vi "RSW_array.vi"() -> ()   [LabVIEW 2015]
doc: "Reading an ini file, sorting using an array, writing sorted data to an ini file"
uses:
  <vilib>/Utility/config.llb/Read Key (String).vi
  <vilib>/Utility/config.llb/Write Key (String).vi
  <vilib>/Utility/config.llb/Write Key (Double).vi
  <vilib>/Utility/config.llb/NI_LVConfig.lvlib
panel:
  out "Sorted":T1(array[cluster])
  out "Unsorted":T1(array[cluster])
  out "error out":errorcluster
  in  "Sorted ini file":path
  in  "The path of the ini file":path
  in  "Cluster":T2
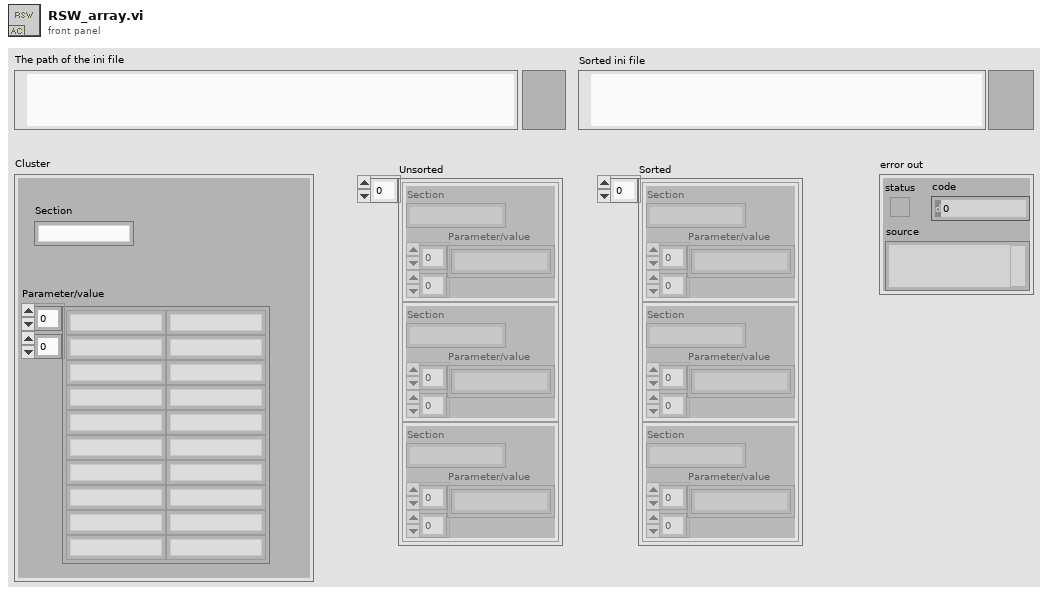
[diagram p1: front panel]
types:
  T1 = cluster{"Section":string, "Parameter/value":string[][]}[]
  T2 = cluster{"Section":string, "Parameter/value":string[][]}
  T3 = typedef "NI_LVConfig.lvlib/Config Data RefNum.ctl" = refnum<k1>
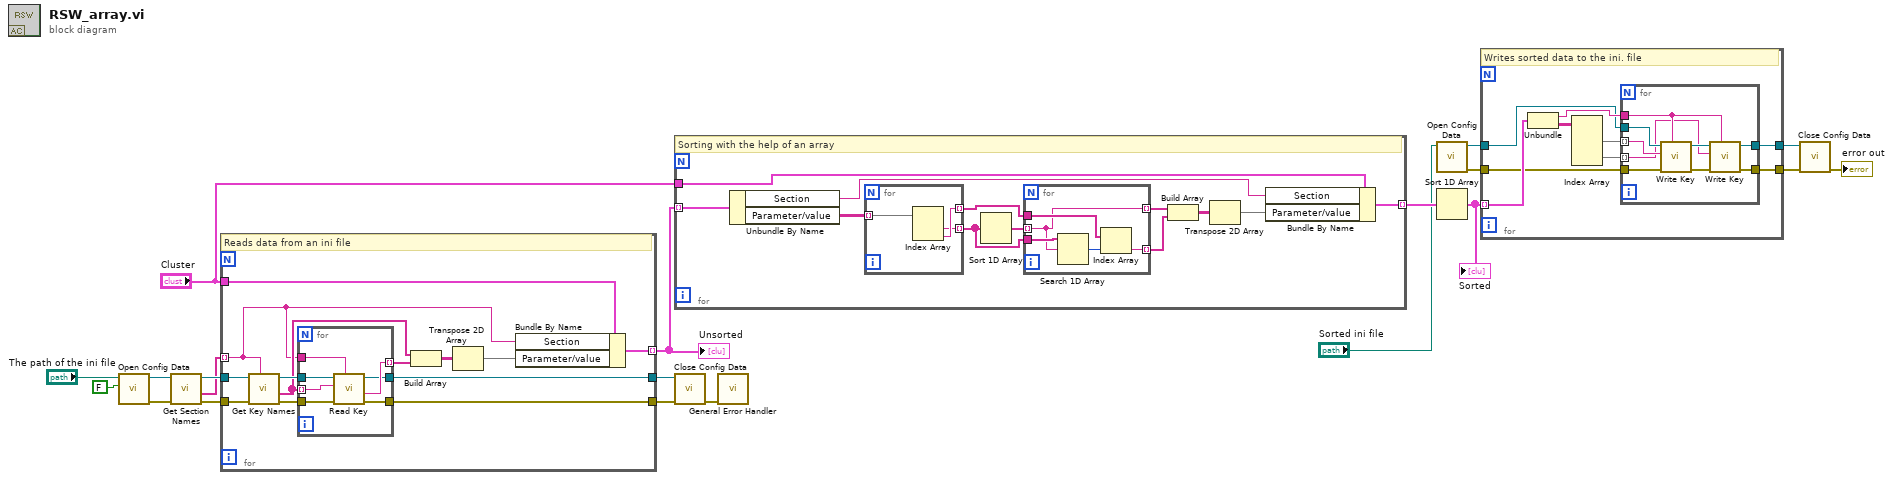
[diagram p0: block diagram]
diagram:
  n1 = call <vilib>:"Open Config Data.vi"("create file if necessary (T)"=FALSE, "configuration file path"="The path of the ini file") -> ("error out"=w19:errorcluster, "refnum"=w20:T3)  [unwired: 7 in, 1 out]
  n2 = call <vilib>:"Get Section Names.vi"("error in (no error)"=w19, "refnum"=w20) -> ("error out"=w17:errorcluster, "section names"=w16:string[], "refnum out"=w18:T3)  [unwired: 7 in]
  n3 = for {
    tunnel: w16 -> [w26] mode=indexing
    tunnel: w18 -> [w32]
    tunnel: w17 -> [w33]
    tunnel: [w25] -> w2 mode=indexing
    tunnel: "Cluster" -> [w24]
    tunnel: [w22] -> w9
    tunnel: [w21] -> w10
    # "Reads data from an ini file"
    n4 = call <vilib>:"Get Key Names.vi"("section"=w26, "error in (no error)"=w33, "refnum"=w32) -> ("error out"=w31:errorcluster, "key names"=w29:string[], "refnum out"=w30:T3)  [unwired: 5 in, 1 out]
    n5 = for {
      tunnel: w26 -> [w40]
      tunnel: w29 -> [w39] mode=indexing
      tunnel: w30 -> [w38]
      tunnel: w31 -> [w37]
      tunnel: [w36] -> w28 mode=indexing
      tunnel: [w35] -> w22
      tunnel: [w34] -> w21
      n6 = call-poly <vilib>:"Read Key.vi"("section"=w40, "error in (no error)"=w37, "key"=w39, "refnum"=w38) -> ("error out"=w35:errorcluster, "value"=w36:string, "refnum out"=w34:T3)  [unwired: 4 in, 1 out]
    }
    n7 = Build Array(w29, w28) -> (w27:string[][])
    n8 = Transpose 2D Array(2D array=w27) -> (transposed array=w23:string[][])
    n9 = Bundle By Name(cluster=w24, "Section"=w26, "Parameter/value"=w23) -> (w25:T2)
  }
  "Unsorted" <- w2
  n10 = for {
    tunnel: w2 -> [w52] mode=indexing
    tunnel: "Cluster" -> [w50]
    tunnel: [w51] -> w12 mode=indexing
    # "Sorting with the help of an array"
    n11 = Unbundle By Name(w52) -> ("Section"=w49:string, "Parameter/value"=w42:string[][])
    n12 = for {
      tunnel: [w55] -> w48 mode=indexing
      tunnel: [w54] -> w46 mode=indexing
      tunnel: w42 -> [w53] mode=indexing
      n13 = Index Array(array=w53) -> (element #1=w54:string, element #2=w55:string)  [unwired: 2 in]
    }
    n14 = Sort 1D Array(array=w46) -> (sorted array=w47:string[])
    n15 = for {
      tunnel: w48 -> [w59]
      tunnel: w47 -> [w56] mode=indexing
      tunnel: w46 -> [w60]
      tunnel: [w57] -> w44 mode=indexing
      tunnel: [w56] -> w43 mode=indexing
      n16 = Search 1D Array(1D array=w60, element=w56) -> (index of element=w58:i32)  [unwired: 1 in]
      n17 = Index Array(array=w59, index=w58) -> (element=w57:string)
    }
    n18 = Build Array(w43, w44) -> (w45:string[][])
    n19 = Transpose 2D Array(2D array=w45) -> (transposed array=w41:string[][])
    n20 = Bundle By Name(cluster=w50, "Section"=w49, "Parameter/value"=w41) -> (w51:T2)
  }
  n21 = call <vilib>:"Close Config Data.vi"("error in (no error)"=w9, "refnum"=w10) -> ("error out"=w11:errorcluster)  [unwired: 8 in, 1 out]
  n22 = call <vilib>:"General Error Handler.vi"("error in (no error)"=w11) -> ()  [unwired: 10 in, 5 out]
  n23 = call <vilib>:"Open Config Data.vi"("configuration file path"="Sorted ini file") -> ("error out"=w7:errorcluster, "refnum"=w8:T3)  [unwired: 8 in, 1 out]
  n24 = Sort 1D Array(array=w12) -> (sorted array=w3:T1)
  "Sorted" <- w3
  n25 = for {
    tunnel: w3 -> [w69] mode=indexing
    tunnel: w8 -> [w66]
    tunnel: w7 -> [w63]
    tunnel: [w62] -> w6
    tunnel: [w61] -> w5
    # "Writes sorted data to the ini. file"
    n26 = Unbundle(w69) -> ("Section"=w67:string, "Parameter/value"=w68:string[][])
    n27 = Index Array(array=w68) -> (element #1=w65:string[], element #2=w64:string[])  [unwired: 4 in]
    n28 = for {
      tunnel: w67 -> [w78]
      tunnel: w66 -> [w77]
      tunnel: w65 -> [w75] mode=indexing
      tunnel: w64 -> [w74] mode=indexing
      tunnel: w63 -> [w73]
      tunnel: [w71] -> w62
      tunnel: [w70] -> w61
      n29 = call-poly <vilib>:"Write Key.vi"("section"=w78, "error in (no error)"=w73, "key"=w75, "refnum"=w77) -> ("error out"=w72:errorcluster, "refnum out"=w76:T3)  [unwired: 5 in, 1 out]
      n30 = call-poly <vilib>:"Write Key.vi"("section"=w78, "error in (no error)"=w72, "key"=w74, "refnum"=w76) -> ("error out"=w71:errorcluster, "refnum out"=w70:T3)  [unwired: 5 in, 1 out]
    }
  }
  n31 = call <vilib>:"Close Config Data.vi"("error in (no error)"=w6, "refnum"=w5) -> ("error out"=→"error out":errorcluster)  [unwired: 8 in, 1 out]
